vi "Load MP3.vi"(8 "error in (no error)":errorcluster, 11 "Path":path) -> (0 "error out":errorcluster, 1 "data":waveform(i16)[](array[waveform]), 2 "Sample Rate (Hz)":u32, 3 "Channels":u32, 5 "Length (Samples)":u64)   [LabVIEW 2019, in "LabVIEW Audio Codecs.lvlib"]
doc: "Loads an MP3 file from disk.\n\n<b>Priority:</b> Background priority (lowest)"
uses:
  LabVIEW Audio Codecs.lvlib
  labview_audio_codecs_x86.dll
  labview_audio_codecs_x64.dll
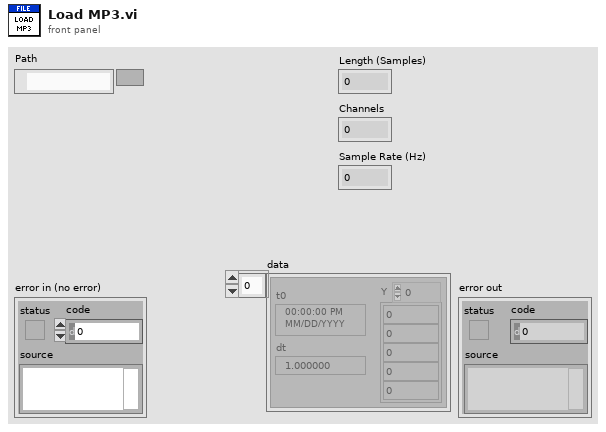
[diagram p1: front panel]
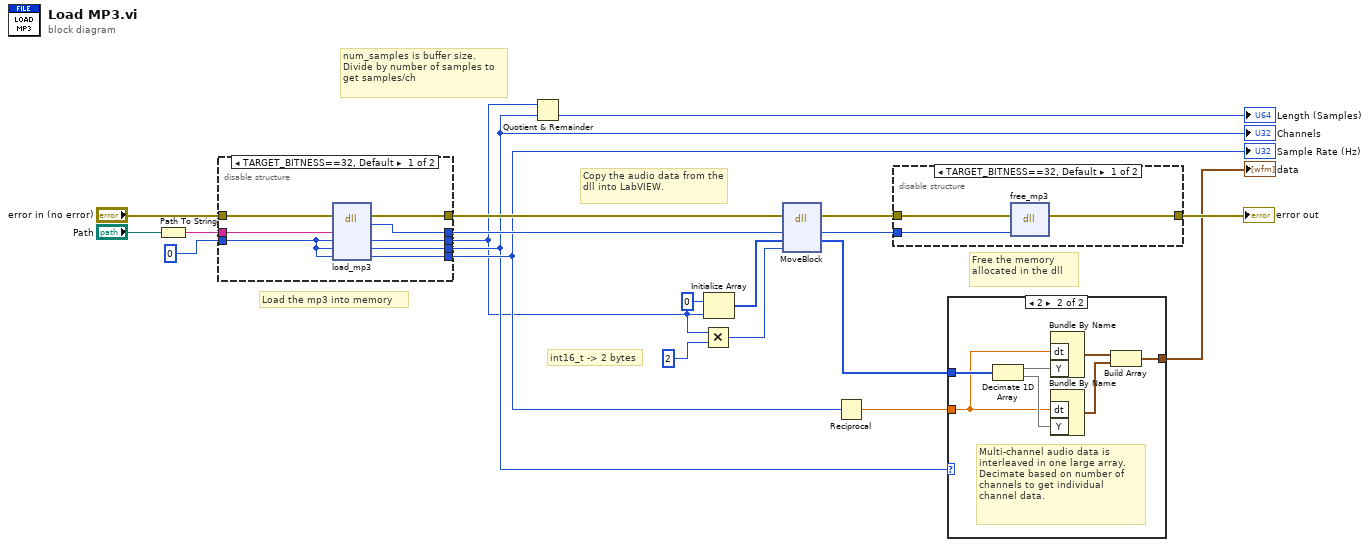
[diagram p0: block diagram]
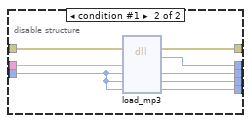
[diagram p2: hidden frame]
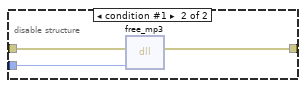
[diagram p3: hidden frame]
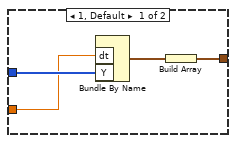
[diagram p4: hidden frame]
diagram:
  # "num_samples is buffer size. Divide by number of samples to get samples/ch"
  # "Free the memory allocated in the dll"
  # "Copy the audio data from the dll into LabVIEW."
  # "Load the mp3 into memory"
  # "int16_t -> 2 bytes"
  n1 = Path To String(path="Path") -> (string=w16:string)
  n2 = disable-structure shown="TARGET_BITNESS==32, Default" {
    disable-tunnel: "error in (no error)" -> [w28 w36]
    disable-tunnel: [w25 w33] -> w1
    disable-tunnel: [w24 w32] -> w3
    disable-tunnel: [w23 w31] -> w5
    disable-tunnel: w16 -> [w21 w29]
    disable-tunnel: [w26 w34] -> w14
    disable-tunnel: [w27 w35] -> w12
    disable-tunnel: 0 ("num_samples") -> [w22 w30]
    frame condition #0 (active) {
      n3 = dll-call lib="C:/github/dataflowg/labview-simcity-2000-toolkit/src/Sound/LabVIEW Audio Codecs/labview_audio_codecs_x86.*" fn="load_mp3"(error in=w28, "file_name"=w21, "num_samples"=w22, "channels"=w22, "sample_rate"=w22) -> (error out=w27:errorcluster, "return type"=w26:i64, "num_samples"=w25:i32, "channels"=w24:i32, "sample_rate"=w23:i32)  [unwired: 3 in, 1 out]
    }
    frame condition #1 {
      n4 = dll-call lib="C:/github/dataflowg/labview-audio-codecs/src/LabVIEW/LabVIEW Audio Codecs/labview_audio_codecs_x64.*" fn="load_mp3"(error in=w36, "file_name"=w29, "num_samples"=w30, "channels"=w30, "sample_rate"=w30) -> (error out=w35:errorcluster, "return type"=w34:i64, "num_samples"=w33:i32, "channels"=w32:i32, "sample_rate"=w31:i32)  [unwired: 3 in, 1 out]
    }
  }
  "Channels" <- w3
  "Sample Rate (Hz)" <- w5
  n5 = Quotient & Remainder(x=w1, y=w3) -> (floor(x/y)=→"Length (Samples)":i32)  [unwired: 1 out]
  n6 = Multiply(x=w1, y=u64 2) -> (x*y=w10:u64)
  n7 = Initialize Array(i16 0 ("num_samples"), w1) -> (w13:i16[])
  n8 = dll-call lib="LabVIEW" fn="MoveBlock"(error in=w12, "Address (Pointer)"=w14, "Destination"=w13, "Size"=w10) -> (error out=w8:errorcluster, "Address (Pointer)"=w9:i64, "Destination"=w7:i16[])  [unwired: 4 in, 1 out]
  n9 = Reciprocal(x=w5) -> (1/x=w4:dbl)
  n10 = disable-structure shown="TARGET_BITNESS==32, Default" {
    disable-tunnel: [w39 w42] -> w19
    disable-tunnel: w9 -> [w38 w41]
    disable-tunnel: w8 -> [w37 w40]
    frame condition #0 (active) {
      n11 = dll-call lib="C:/github/dataflowg/labview-simcity-2000-toolkit/src/Sound/LabVIEW Audio Codecs/labview_audio_codecs_x86.*" fn="free_mp3"(error in=w37, "Address (Pointer)"=w38) -> (error out=w39:errorcluster)  [unwired: 4 in, 1 out]
    }
    frame condition #1 {
      n12 = dll-call lib="C:/github/dataflowg/labview-audio-codecs/src/LabVIEW/LabVIEW Audio Codecs/labview_audio_codecs_x64.*" fn="free_mp3"(error in=w40, "Address (Pointer)"=w41) -> (error out=w42:errorcluster)  [unwired: 4 in, 1 out]
    }
  }
  "error out" <- w19
  n13 = case shown="2" w3 {
    tunnel: w7 -> [w46 w53]
    tunnel: [w45 w48] -> w17
    tunnel: w4 -> [w43 w47]
    frame 1, Default {
      n14 = Bundle By Name("dt"=w43, "Y"=w46) -> (w44:waveform(i16))  [unwired: 1 in]
      n15 = Build Array(w44) -> (w45:waveform(i16)[])
    }
    frame 2 {
      # "Multi-channel audio data is interleaved in one large array. Decimate based on number of channels to get individual channel data."
      n16 = Decimate 1D Array(w53) -> (w52:i16[], w51:i16[])
      n17 = Bundle By Name("dt"=w47, "Y"=w52) -> (w50:waveform(i16))  [unwired: 1 in]
      n18 = Bundle By Name("dt"=w47, "Y"=w51) -> (w49:waveform(i16))  [unwired: 1 in]
      n19 = Build Array(w50, w49) -> (w48:waveform(i16)[])
    }
  }
  "data" <- w17
